vi "ButtonDisable.vi"(8 "Clear Display Button Reference":refnum<vi>, 11 "Preview Button Reference":refnum<vi>) -> ()   [LabVIEW 2014]
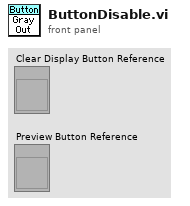
[diagram p1: front panel]
types:
  T1 = enum8{"Enabled", "Disabled", "Disabled and Grayed Out"}
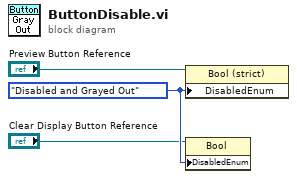
[diagram p0: block diagram]
diagram:
  w3 = T1."Disabled and Grayed Out" ("Disabled")
  n1 = property on="Property Node" class="Bool (strict)"(reference="Preview Button Reference", "DisabledEnum"=w3) -> ()  [unwired: 1 in, 2 out]
  n2 = property on="Property Node" class="Bool"(reference="Clear Display Button Reference", "DisabledEnum"=w3) -> ()  [unwired: 1 in, 2 out]
